vi "JSON_Mult_Read.vi"(2 "Json File Path":path, 5 "ERD Data Out":cluster{"ERD Number":u16, "Data":string}[](array[cluster]) {"ERD Number" format="%.0x"}, 11 "error in":errorcluster) -> (6 "Array":cluster{"ERD Number":u16, "Data":string}[](array[cluster]), 15 "error out":errorcluster)   [LabVIEW 2021]
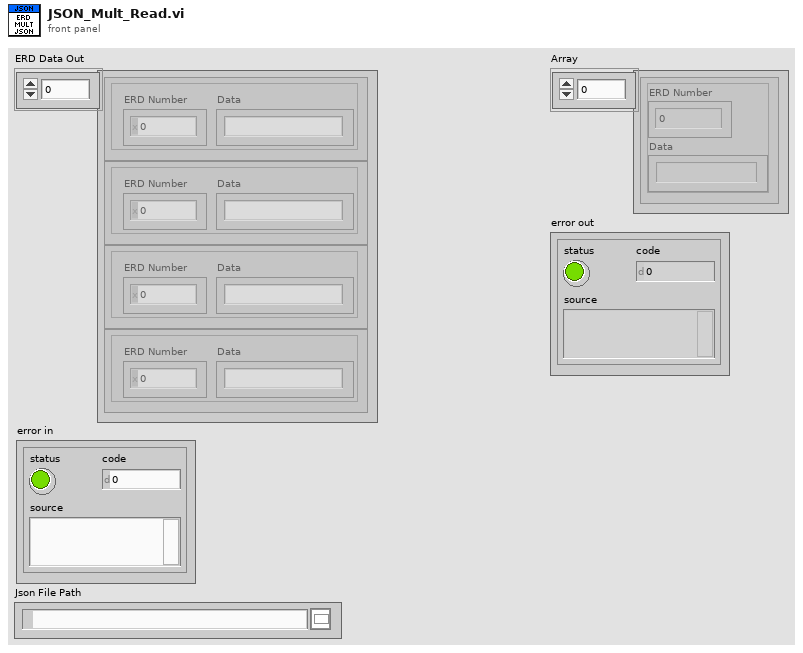
[diagram p1: front panel]
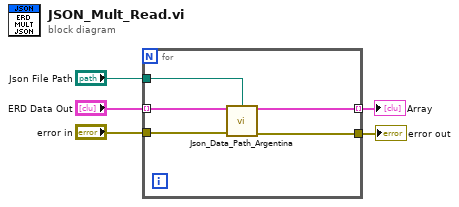
[diagram p0: block diagram]
diagram:
  n1 = for {
    tunnel: "ERD Data Out" -> [w10] mode=indexing
    tunnel: [w9] -> w4 mode=indexing
    tunnel: "error in" -> [w8]
    tunnel: [w7] -> w2
    tunnel: "Json File Path" -> [w6]
    n2 = call "Json_Data_Path_Argentina.vi"("ERD Cluster"=w10, "Json File Path"=w6, "error in"=w8) -> ("ERD JSON"=w9:cluster{"ERD Number":u16, "Data":string}, "error out"=w7:errorcluster)  [unwired: 11 in]
  }
  "Array" <- w4
  "error out" <- w2
